vi "Indruder.vi"() -> ()   [LabVIEW 2020]
uses:
  <vilib>/MakerHub/LINX/Public/Utilities/Open Serial.vi
  <vilib>/httpClient/LabVIEWHTTPClient.lvlib
  <vilib>/MakerHub/LINX/Public/Sensors/Distance/Ultrasonic/Ultrasonic.lvlib
  <vilib>/MakerHub/LINX/LMH-LINX.lvlib
panel:
  out "Error Out":errorcluster
  out "Centimeters":dbl
  in  "System Armed?":bool
  out "Boolean":bool
  out "Iteration":i32
  out "Present (s)":dbl
  out "Elapsed Time (s)":dbl
  in  "stop":bool
  out "INTRUDER ALERT!":bool
  in  "Simulated Capacitive Sensor":bool
  in  "Simulated PIR Sensor":bool
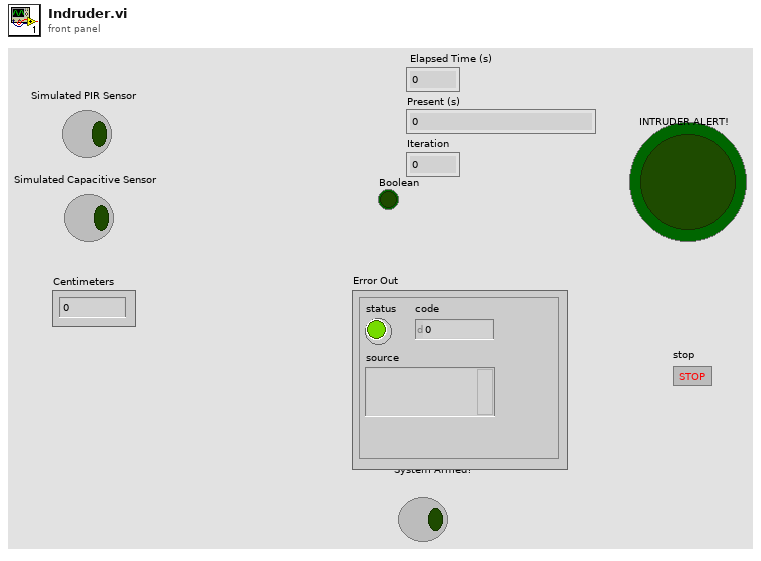
[diagram p1: front panel]
types:
  T1 = typedef "LMH-LINX.lvlib/LINX Ref.ctl" = cluster{"IO":T2, "Interface":T3, "LINX Device Config":T4}
  T2 = typedef "LMH-LINX.lvlib/Platform.ctl" = enum16{"Remote", "Local"}
  T3 = typedef "LMH-LINX.lvlib/Interface.ctl" = enum16{"Serial", "TCP"}
  T4 = typedef "LMH-LINX.lvlib/Device.lvlib/LINX Device Config.ctl" = cluster{"Interface":T3, "COM Port":refnum<visa-resource-name>, "TCP Configuration":T5, "Device Family":u8, "Device ID":u8, "Device Name":string, "TCP Ref":refnum<k5>, "Channels":T6}
  T5 = typedef "LMH-LINX.lvlib/Device.lvlib/TCP Config.ctl" = cluster{"IP Address":string, "Port":u16}
  T6 = typedef "LMH-LINX.lvlib/Channels.ctl" = cluster{"DI":u8[], "DO":u8[], "AI":u8[], "AO":u8[], "PWM":u8[], "QE":u8[], "UART":u8[], "I2C 2":u8[], "SPI":u8[], "CAN":u8[], "Servo":u8[], "AI Ref (V)":dbl, "AI Resolution (Bits)":u8, "AO Ref (V)":dbl, "AO Resolution (Bits)":u8}
  T7 = typedef "LabVIEWHTTPClient.lvlib/ClientHandle.ctl" = refnum<k1>
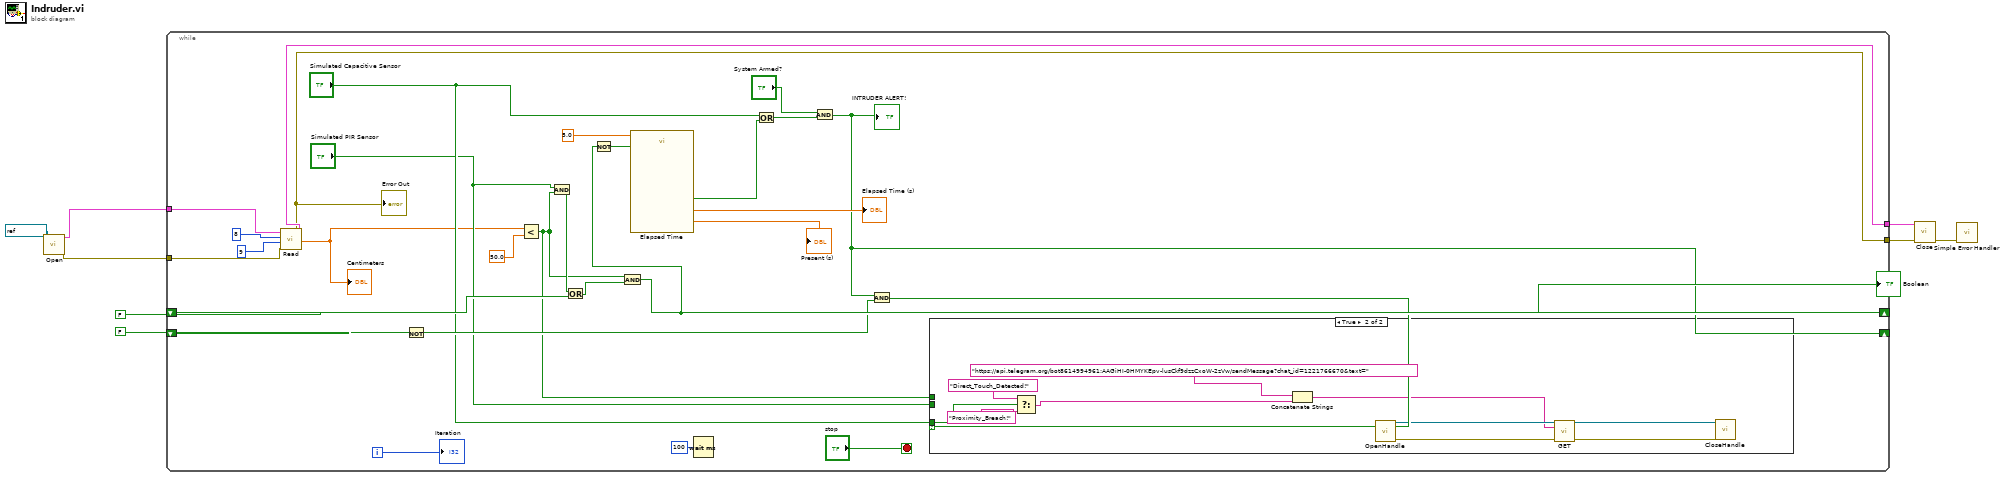
[diagram p0: block diagram]
diagram:
  n1 = call-poly <vilib>:"Open.vi"("Serial Port"=refnum<visa-resource-name> "COM4") -> ("Error Out"=w5:errorcluster, "LINX Resource"=w6:T1)  [unwired: 8 in, 1 out]
  n2 = while {
    shift-right: [w32] -> w8
    shift-left: FALSE -> [w31]
    shift-right: [w20] -> _
    shift-left: FALSE -> [w23]
    tunnel: w6 -> [w15]
    tunnel: w5 -> [w14]
    tunnel: [w12] -> w4
    tunnel: [w13] -> w3
    i -> [w27]
    stop <- "stop" stop-if-true
    n3 = call <vilib>:"Read.vi"("Error In"=w14, "DO Channel"=u8 9, "DI Channel"=u8 8, "LINX Resource"=w15) -> ("Error Out"=w12:errorcluster, "Centimeters"=w16:dbl, "LINX Resource"=w13:T1)  [unwired: 4 in, 1 out]
    "Centimeters" <- w16
    "Error Out" <- w12
    n4 = Not(x=w23) -> (.not. x?=w22:bool)
    n5 = Less?(x=w16, y=50.0) -> (x < y?=w17:bool)
    n6 = And(x="Simulated PIR Sensor", y=w17) -> (x .and. y?=w34:bool)
    n7 = Or(x=w34, y=w31) -> (x .or. y?=w36:bool)
    n8 = And(x=w17, y=w36) -> (x .and. y?=w32:bool)
    n9 = Not(x=w32) -> (.not. x?=w26:bool)
    n10 = call "Elapsed Time"("Time Target (s)"=5.0, "Reset"=w26) -> ("Present (s)"=→"Present (s)":dbl, "Elapsed Time (s)"=→"Elapsed Time (s)":dbl, "Time has Elapsed"=w33:bool)  [unwired: 10 in, 5 out]
    n11 = Wait (ms)(milliseconds to wait=u32 100) -> ()  [unwired: 1 out]
    n12 = Or(x="Simulated Capacitive Sensor", y=w33) -> (x .or. y?=w25:bool)
    n13 = And(x="System Armed?", y=w25) -> (x .and. y?=w20:bool)
    "INTRUDER ALERT!" <- w20
    n14 = And(x=w20, y=w22) -> (x .and. y?=w21:bool)
    n15 = case shown="True" w21 {
      tunnel: "Simulated Capacitive Sensor" -> [_ w40]
      tunnel: "Simulated PIR Sensor" -> [_ _]
      tunnel: w17 -> [_ _]
      frame False {
      }
      frame True {
        n16 = Select(t="Direct_Touch_Detected!", s=w40, f="Proximity_Breach!") -> (s? t:f=w43:string)
        n17 = Concatenate Strings("https://api.telegram.org/bot8614994961:AAGiHI-0HMYKEpv-lusCkf9dzzCxoW-2zVw/sendMessage?chat_id=1221766670&text=", w43) -> (w39:string)
        n18 = call <vilib>:"OpenHandle.vi"() -> ("client handle out"=w48:T7, "error out"=w47:errorcluster)  [unwired: 14 in]
        n19 = call <vilib>:"GET.vi"("client handle"=w48, "url"=w39, "error in (no error)"=w47) -> ("client handle out"=w46:T7, "error out"=w45:errorcluster)  [unwired: 9 in, 2 out]
        n20 = call <vilib>:"CloseHandle.vi"("client handle"=w46, "error in (no error)"=w45) -> ()  [unwired: 13 in, 1 out]
      }
    }
    "Iteration" <- w27
  }
  "Boolean" <- w8
  n21 = call <vilib>:"Close.vi"("Error In"=w4, "LINX Resource"=w3) -> ("Error Out"=w2:errorcluster)  [unwired: 9 in]
  n22 = call <vilib>:"Simple Error Handler.vi"("error in (no error)"=w2) -> ()  [unwired: 4 in, 5 out]
